vi "MissionLocation.vi"(8 "Error In":errorcluster, 11 "GoTo in":refnum<class "GoTo.lvclass">) -> (0 "Error Out":errorcluster, 2 "element":T1 {"North" format="%#_10f"; "East" format="%#_8f"}, 3 "GoTo out":refnum<class "GoTo.lvclass">)   [LabVIEW 2013, in "GoTo.lvclass"]
uses:
  GoTo.lvclass
  Data/TypeDefs/UTM Location.ctl
  GenericMission/GenericMission.lvclass
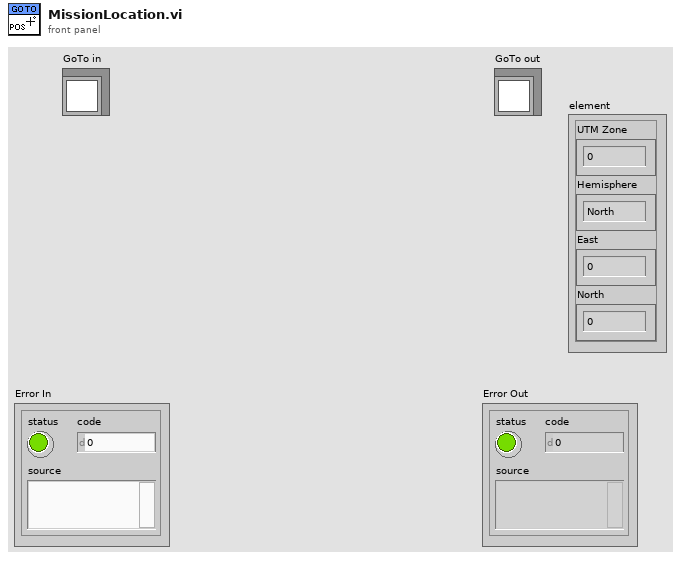
[diagram p1: front panel]
types:
  T1 = typedef "UTM Location.ctl" = cluster{"UTM Zone":dbl, "Hemisphere":enum16{"North", "South"}, "East":dbl, "North":dbl}
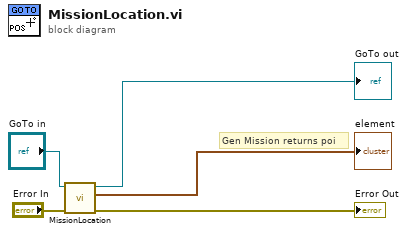
[diagram p0: block diagram]
diagram:
  # "Gen Mission returns poi"
  n1 = call-parent "MissionLocation.vi"("Error In"="Error In", "GenericMission in"="GoTo in") -> ("Error Out"=→"Error Out":errorcluster, "element"=→"element":T1, "GenericMission out"=→"GoTo out":refnum<class "GoTo.lvclass">)  [unwired: 7 in]
